vi "ConvertUnitValueToDouble.vi"(11 "value":string) -> (3 "result":dbl format="%#_6f")   [LabVIEW 2018, in "Library-DataConvert.lvlib"]
uses:
  Library-DataConvert.lvlib
  <vilib>/regexp/Match Regular Expression.xnode
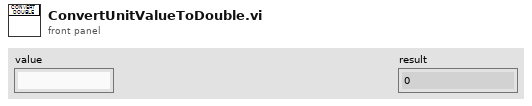
[diagram p1: front panel]
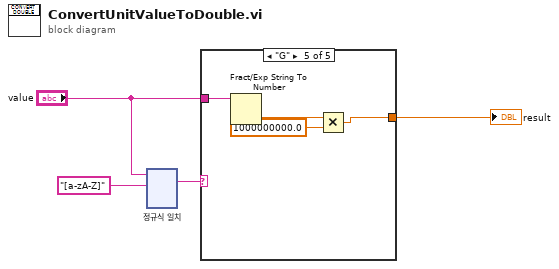
[diagram p0: block diagram]
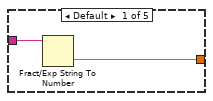
[diagram p2: hidden frame]
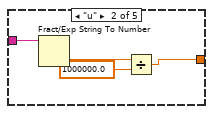
[diagram p3: hidden frame]
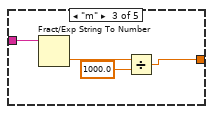
[diagram p4: hidden frame]
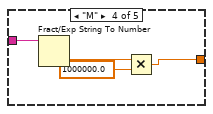
[diagram p5: hidden frame]
diagram:
  n1 = xnode "정규식 일치"("입력 문자열"="value", "정규식"="[a-zA-Z]") -> ("전체 일치 구문"=w3:string)  [unwired: 4 in, 4 out]
  n2 = case shown="\"G\"" w3 {
    tunnel: "value" -> [w6 w10 w14 w18 w22]
    tunnel: [w5 w7 w11 w15 w19] -> w1
    frame Default {
      n3 = Fract/Exp String To Number(string=w6) -> (number=w5:dbl)  [unwired: 3 in, 1 out]
    }
    frame "u" {
      n4 = Fract/Exp String To Number(string=w10) -> (number=w9:dbl)  [unwired: 3 in, 1 out]
      n5 = Divide(x=w9, y=1000000.0) -> (x/y=w7:dbl)
    }
    frame "m" {
      n6 = Fract/Exp String To Number(string=w14) -> (number=w13:dbl)  [unwired: 3 in, 1 out]
      n7 = Divide(x=w13, y=1000.0) -> (x/y=w11:dbl)
    }
    frame "M" {
      n8 = Fract/Exp String To Number(string=w18) -> (number=w17:dbl)  [unwired: 3 in, 1 out]
      n9 = Multiply(x=w17, y=1000000.0) -> (x*y=w15:dbl)
    }
    frame "G" {
      n10 = Fract/Exp String To Number(string=w22) -> (number=w21:dbl)  [unwired: 3 in, 1 out]
      n11 = Multiply(x=w21, y=1000000000.0) -> (x*y=w19:dbl)
    }
  }
  "result" <- w1
